vi "SafeIntakeMode.vi"() -> (0 "Rollers Active?":bool, 1 "Angle Power":dbl, 3 "Roller Power":dbl)   [LabVIEW 2015]
uses:
  Common Code/Intake States.ctl
  Common Code/Intake Commands.ctl
  Robot Global Data.vi
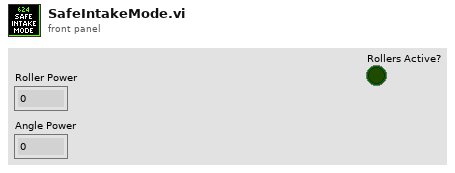
[diagram p1: front panel]
types:
  T1 = typedef "Intake States.ctl" = enum16{"Idle", "Set roller speed", "Move to angle"}
  T2 = typedef "Dashboard Control Data.ctl" = cluster{"Shooter Presets":T3, "Encoder Control":T5, "Steer PID output":cluster{"output high":dbl, "output low":dbl}, " Steer PID gains":cluster{"proportional gain (Kc)":dbl, "integral time (Ti, min)":dbl, "derivative time (Td, min)":dbl}, "Drivetrain Settings":T6, "Vision Packet":T7, "Dashboard Drivetrain Command":T8, "Info/Command Cluster":T10, "Ball Vision Packet":T11, "Intake Presets":T13, "Intake Encoder Control":T15, "Climb Presets":T16, "Goal Output Range":cluster{"output high":dbl, "output low":dbl}}
  T3 = typedef "Shooter Presets.ctl" = cluster{"Batter Shot":T4, "Low Bar Curve Shot":T4, "Deep Middle Shot":T4, "Manual Shot":T4, "Left Ticks Per Rotation":dbl, "Right Ticks Per Rotation":dbl, "Low Bar Shot":T4, "Shooter RPM Tolerance":dbl, "IIR Filter Power":dbl, "Trigger Power":dbl, "Fire from Load Delay":i32, "Angle Pot M":dbl, "Angle Pot B":dbl, "Shooter Deck Length":dbl, "String Pot Dist From Pivot":dbl, "Angle PID gains":cluster{"proportional gain (Kc)":dbl, "integral time (Ti, min)":dbl, "derivative time (Td, min)":dbl}, "Angle Motor Output Range":cluster{"output high":dbl, "output low":dbl}, "Shooter Angle Tolerance":dbl, "Vision Shoot x^2":dbl, "Vision Shoot x":dbl, "Dist from Axis Cam to Pivot":dbl, "High Goal Center Height":dbl, "Feed Forward Max Accel":dbl, "Feed Forward Kv":dbl, "Backwards Trigger":dbl, "Shot Finish Delay (ms)":dbl, "Angle Max Current":dbl, "Angle Current Trip Time":dbl, "Shooter Intake Angle":dbl, "Vision Shoot c":dbl, "Reset?":bool}
  T4 = typedef "Shot Presets.ctl" = cluster{"Left Wheel RPM":dbl, "Right Wheel RPM":dbl, "Angle":dbl}
  T5 = typedef "Encoder Control.ctl" = cluster{"Right Tick Constant":dbl, "Left Tick Constant":dbl, "Reset?":bool, "Y Dist":cluster{"PID gains":cluster{"proportional gain (Kc)":dbl, "integral time (Ti, min)":dbl, "derivative time (Td, min)":dbl}}, "Y Stop Thresh":dbl, "Y Stop Speed":dbl}
  T6 = typedef "Drivetrain Settings.ctl" = cluster{"Gyro Tolerance":dbl, "Throttle Ramp (ms)":dbl, "Angular rate compensation":bool, "Throttle to Rate Scale":dbl, "Rate compensation gain":dbl, "Kv":dbl, "Ka":dbl, "Feed Forward P":dbl, "Feed Forward D":dbl, "Goal Vision PID gains":cluster{"proportional gain (Kc)":dbl, "integral time (Ti, min)":dbl, "derivative time (Td, min)":dbl}, "Goal Detection Window":dbl}
  T7 = typedef "Goal Vision Packet.ctl" = cluster{"Distance":dbl, "Center X":dbl, "Center Y":dbl, "Found Target?":bool}
  T8 = typedef "Dashboard Drivetrain Command.ctl" = cluster{"Drivetrain Vision":T9}
  T9 = typedef "Drivetrain Vision.ctl" = cluster{"Goal Window":dbl, "Ball Window":dbl}
  T10 = typedef "Ball Tracking Command Cluster.ctl" = cluster{"Distance to Ball":dbl, "Desired Angle":dbl, "Command":enum16{"Turn to Ball", "Turn to Angle", "Get Distance"}, "Pixels from Center":dbl}
  T11 = typedef "Ball Vision Packet.ctl" = cluster{"Ball Detected?":bool, "Distance to Ball":dbl, "Desired Angle":dbl, "Pixels from Center":dbl, "Tracking mode":T12}
  T12 = typedef "Tracking Mode.ctl" = enum16{"Turn to Ball", "Turn to Angle"}
  T13 = typedef "Intake Presets.ctl" = cluster{"Intake Speed":dbl, "Outake Speed":dbl, "Low Height":dbl, "Half Height":dbl, "Full Height":dbl, "Angle Speed":dbl, "Fast Angle":dbl, "Encoder Scale Factor":dbl, "Load Height":dbl, "Output Range":T14, "PID Params":cluster{"PID gains":cluster{"proportional gain (Kc)":dbl, "integral time (Ti, min)":dbl, "derivative time (Td, min)":dbl}}, "Rotation Power Max/Min":dbl, "MaxCurrent":dbl, "Intake Trip Time":dbl, "Idle Height":dbl, "Max Height":dbl, "Reset Encoders?":bool}
  T14 = typedef "Drivetrain Output Range.ctl" = cluster{"output high":dbl, "output low":dbl}
  T15 = typedef "IntakeEcoderControl.ctl" = cluster{"Arm Tick Constant":dbl, "Reset?":bool, "Y Dist":cluster{"PID gains":cluster{"proportional gain (Kc)":dbl, "integral time (Ti, min)":dbl, "derivative time (Td, min)":dbl}}, "Y Stop Thresh":dbl, "Y Stop Speed":dbl}
  T16 = typedef "Climb Presets.ctl" = cluster{"Pull Power":dbl, "Unpin Power":dbl, "Time to Hold":dbl}
  T17 = typedef "Intake Commands Cluster.ctl" = cluster{"Intake Commands":T18, "Intake Mode":T19, "Override IR":bool}
  T18 = typedef "Intake Commands.ctl" = enum16{"Unload", "Load", "Pull up", "Drop low", "Idle", "Lift Half"}
  T19 = typedef "Intake Mode.ctl" = enum16{"Safe", "Auto", "Manual"}
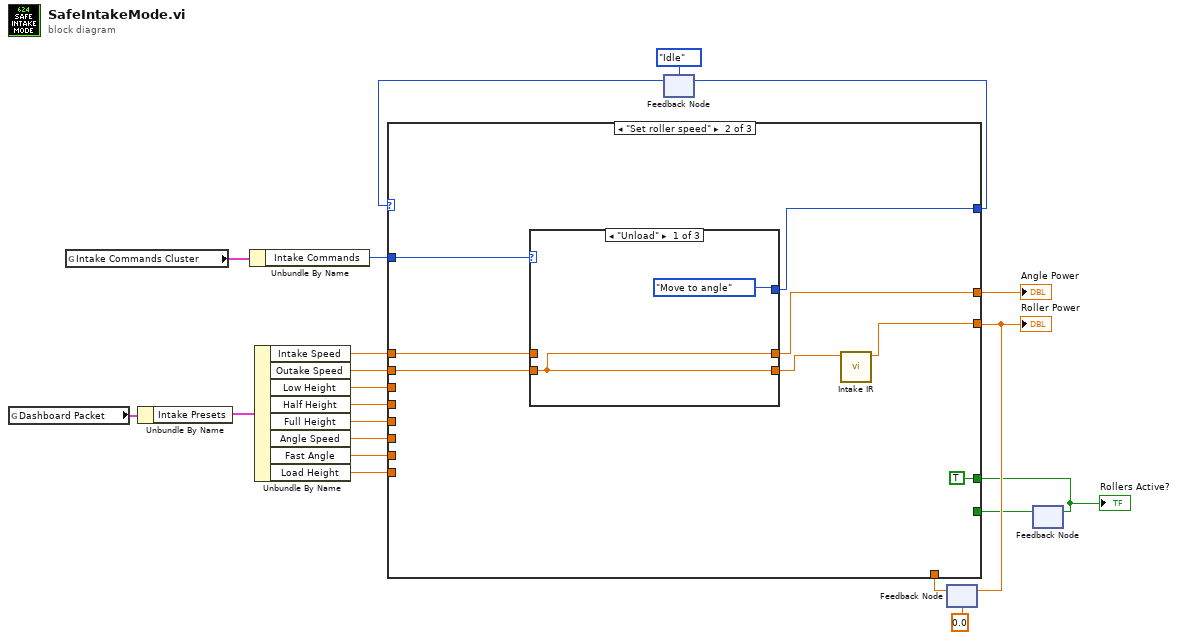
[diagram p0: block diagram]
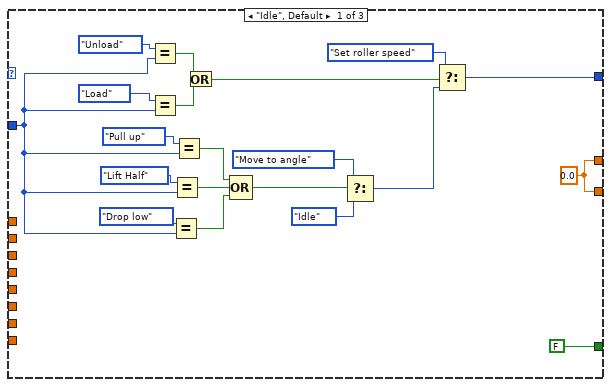
[diagram p2: hidden frame]
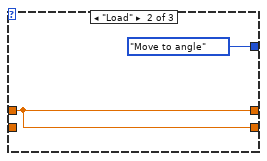
[diagram p3: hidden frame]
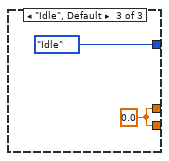
[diagram p4: hidden frame]
diagram:
  n1 = global read "Robot Global Data.vi" "Dashboard Packet"() -> (w21:T2)
  n2 = global read "Robot Global Data.vi" "Intake Commands Cluster"() -> (w7:T17)
  n3 = Unbundle By Name(w21) -> ("Intake Presets"=w20:T13)
  n4 = Unbundle By Name(w7) -> ("Intake Commands"=w12:T18)
  n5 = Unbundle By Name(w20) -> ("Intake Speed"=w19:dbl, "Outake Speed"=w18:dbl, "Low Height"=w17:dbl, "Half Height"=w16:dbl, "Full Height"=w15:dbl, "Angle Speed"=w14:dbl, "Fast Angle"=w13:dbl, "Load Height"=w6:dbl)
  n6 = feedback #1(Intake_States."Idle" ("Intake States")) -> (w11:T1)
  n7 = feedback #2(0.0 ("Intake Speed")) -> (w8:dbl)
  n8 = feedback #3() -> (w1:bool)  [unwired: 1 in]
  n9 = case shown="\"Set roller speed\"" w11 {
    tunnel: w19 -> [_ w49 _]
    tunnel: w18 -> [_ w48 _]
    tunnel: w17 -> [_ _ _]
    tunnel: w16 -> [_ _ _]
    tunnel: w15 -> [_ _ _]
    tunnel: w14 -> [_ _ _]
    tunnel: w13 -> [_ _ _]
    tunnel: w12 -> [w23 w46 _]
    tunnel: [w25 w47 _] -> w10
    tunnel: [w24 w42 w57] -> w4
    tunnel: w8 -> [_ _ w57]
    tunnel: w6 -> [_ _ _]
    tunnel: [w24 w45 _] -> w5
    tunnel: [FALSE TRUE w56] -> w2
    tunnel: w1 -> [_ _ w56]
    frame "Idle", Default {
      w24 = 0.0
      n10 = Equal?(x=Intake_Commands."Unload" ("Intake Commands"), y=w23) -> (x = y?=w39:bool)
      n11 = Equal?(x=Intake_Commands."Load" ("Intake Commands"), y=w23) -> (x = y?=w38:bool)
      n12 = Equal?(x=Intake_Commands."Drop low" ("Intake Commands"), y=w23) -> (x = y?=w32:bool)
      n13 = Equal?(x=Intake_Commands."Lift Half" ("Intake Commands"), y=w23) -> (x = y?=w33:bool)
      n14 = Equal?(x=Intake_Commands."Pull up" ("Intake Commands"), y=w23) -> (x = y?=w34:bool)
      n15 = Or(x=w39, y=w38) -> (x .or. y?=w31:bool)
      n16 = Compound Arithmetic op=OR(w34, w33, w32) -> (w29:bool)
      n17 = Select(t=Intake_States."Move to angle" ("Intake States"), s=w29, f=Intake_States."Idle" ("Intake States")) -> (s? t:f=w26:T1)
      n18 = Select(t=Intake_States."Set roller speed" ("Intake States"), s=w31, f=w26) -> (s? t:f=w25:T1)
    }
    frame "Set roller speed" {
      n19 = case shown="\"Unload\"" w46 {
        tunnel: w49 -> [_ w52 _]
        tunnel: w48 -> [w50 _ _]
        tunnel: [w50 w52 w54] -> w43
        tunnel: [Intake_States."Move to angle" ("Intake States") Intake_States."Move to angle" ("Intake States") Intake_States."Idle" ("Intake States")] -> w47
        tunnel: [w50 w52 w54] -> w45
        frame "Unload" {
        }
        frame "Load" {
        }
        frame "Idle", Default {
          w54 = 0.0 ("Intake Speed")
        }
      }
      n20 = call "Intake IR.vi"("Speed"=w43) -> ("Speeeeeeed"=w42:dbl)  [unwired: 10 in]
    }
    frame "Move to angle" {
    }
  }
  "Angle Power" <- w5
  "Roller Power" <- w4
  "Rollers Active?" <- w2
  n21 = feedback-in #1(w10) -> ()
  n22 = feedback-in #2(w4) -> ()
  n23 = feedback-in #3(w2) -> ()
